vi "modelFrameworkVersion.vi"() -> (3 "Version":T1)   [LabVIEW 2019]
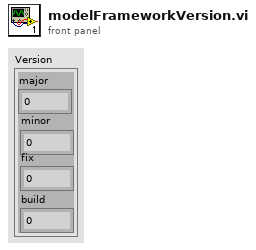
[diagram p1: front panel]
types:
  T1 = cluster{"major":u32, "minor":u32, "fix":u32, "build":u32}
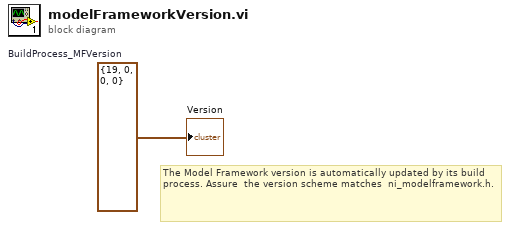
[diagram p0: block diagram]
diagram:
  w1 = T1 {"major"=19, "minor"=0, "fix"=0, "build"=0}  # BuildProcess_MFVersion
  # "The Model Framework version is automatically updated by its build process. Assure  the version scheme matches  ni_modelframework.h."
  "Version" <- w1
